vi "LS218_WRITE_TYPE_SONDES.vi"(4 "entrée d'erreur (pas d'erreur)":errorcluster, 5 "A ou B":string, 6 "Input_type":u16(ring)=6 items=["aucune", "DT-470 (diode)", "DT-500 (diode)", "CTI (diode)", "DT- 670 (diode)", "Cernox", "Pt100", "Pt1000"], 7 "Refnum VISA en entrée":refnum<visa-resource-name>) -> (0 "sortie d'erreur":errorcluster, 3 "Nom de ressource VISA en sortie":refnum<visa-resource-name>)   [LabVIEW 2016]
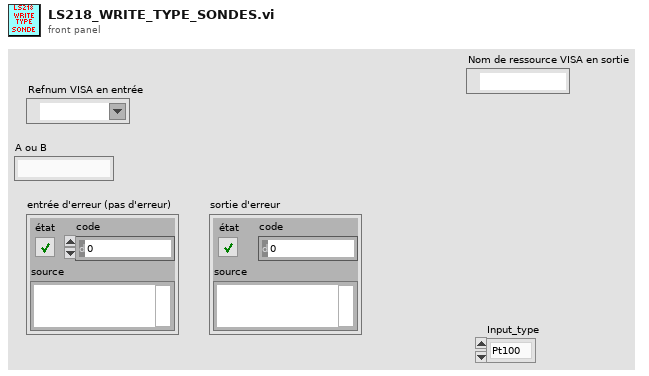
[diagram p1: front panel]
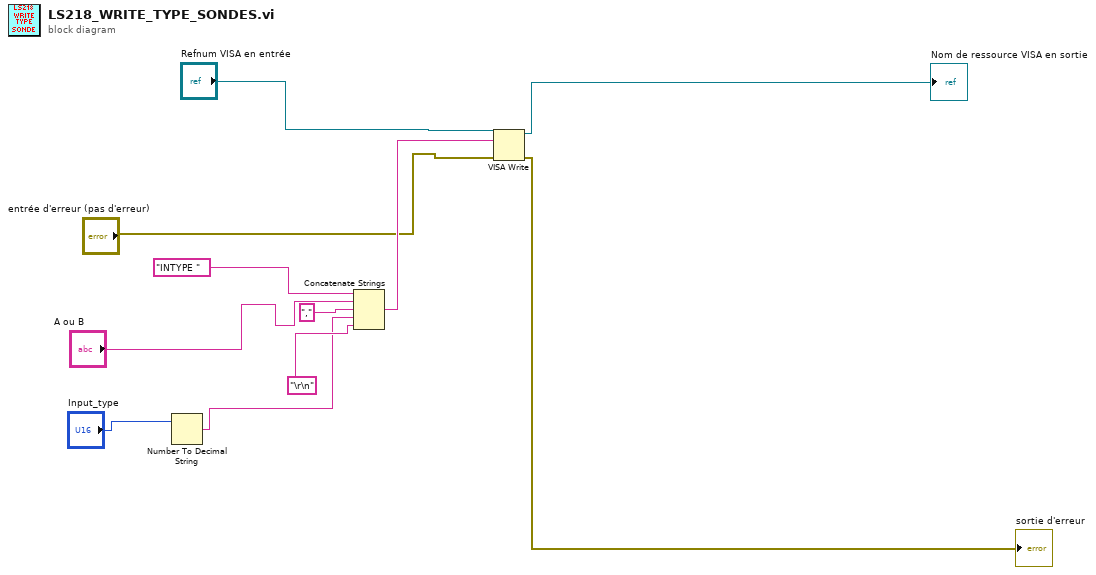
[diagram p0: block diagram]
diagram:
  n1 = Number To Decimal String ("Nombre en chaîne décimale")(number="Input_type") -> (decimal integer string=w9:string)  [unwired: 1 in]
  n2 = Concatenate Strings("INTYPE " ("chaîne"), "A ou B", "," ("chaîne"), w9, "\r\n" ("chaîne")) -> (w5:string)
  n3 = VISA Write(VISA resource name="Refnum VISA en entrée", write buffer=w5, error in (no error)="entrée d'erreur (pas d'erreur)") -> (VISA resource name out=→"Nom de ressource VISA en sortie":refnum<visa-resource-name>, error out=→"sortie d'erreur":errorcluster)  [unwired: 1 out]
